vi "LVSPrtHlpHD.vi"(9 "Help?":string, 11 "VISA resource name":refnum<visa-resource-name>) -> (0 "error?":bool, 2 "string read":string)   [LabVIEW 2017]
uses:
  <vilib>/Utility/error.llb/DialogType.ctl
  Program Files (x86)/National Instruments/LabVIEW 2017/instr.lib/lvserial/lvserial.lvlib
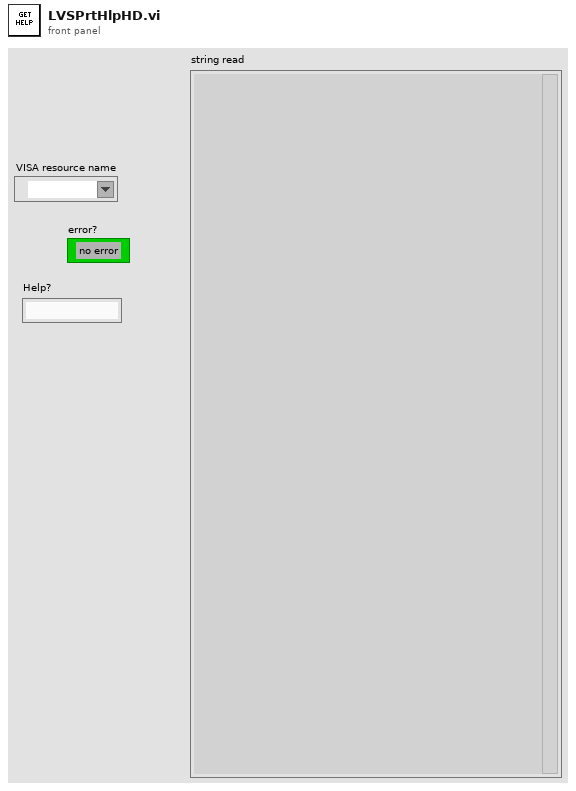
[diagram p1: front panel]
types:
  T1 = typedef "DialogType.ctl" = u16
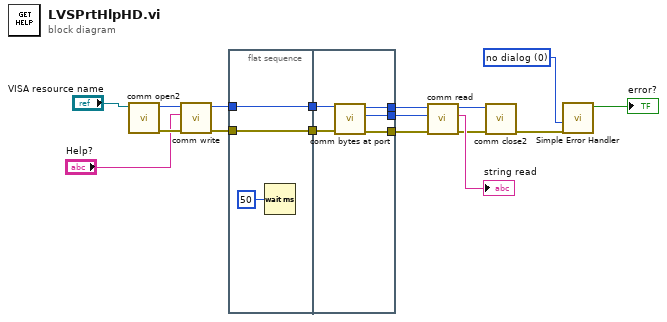
[diagram p0: block diagram]
diagram:
  w4 = T1 0 items=["no dialog", "OK message", "continue or stop message", "OK message + warnings", "continue/stop + warnings"] ("type of dialog (OK msg:1)")
  n1 = call "comm open2.vi"("Comm Port Name"="VISA resource name") -> ("error out"=w14:errorcluster, "Comm Handle"=w13:u32)  [unwired: 4 in, 1 out]
  n2 = call "comm write.vi"("error in (no error)"=w14, "string to write"="Help?", "Comm Handle"=w13) -> ("error out"=w8:errorcluster, "dup Comm Handle"=w9:u32)  [unwired: 6 in, 1 out]
  n3 = flat-sequence {
    tunnel: w9 -> [w19]
    tunnel: w8 -> [w18]
    tunnel: [w19] -> w11
    tunnel: [w18] -> w10
    tunnel: [w25] -> w12
    tunnel: w11 -> [w24]
    tunnel: w10 -> [w23]
    tunnel: [w22] -> w6
    tunnel: [w21] -> w5
    frame #0 {
      n4 = Wait (ms)(milliseconds to wait=u32 50) -> ()  [unwired: 1 out]
    }
    frame #1 {
      n5 = call "comm bytes at port.vi"("error in (no error)"=w23, "Comm Handle"=w24) -> ("error out"=w21:errorcluster, "bytes at port"=w25:u32, "dup Comm Handle"=w22:u32)  [unwired: 7 in]
    }
  }
  n6 = call "comm read.vi"("error in (no error)"=w5, "requested byte count"=w12, "Comm Handle"=w6) -> ("error out"=w7:errorcluster, "string read"=→"string read":string, "dup Comm Handle"=w16:u32)  [unwired: 5 in, 1 out]
  n7 = call "comm close2.vi"("error in (no error)"=w7, "Comm Handle"=w16) -> ("error out"=w2:errorcluster)  [unwired: 5 in]
  n8 = call <vilib>:"Simple Error Handler.vi"("type of dialog (OK msg:1)"=w4, "error in (no error)"=w2) -> ("error?"=→"error?":bool)  [unwired: 7 out]
